vi "InitRegisterLambdaSIM.vi"(8 "error in":errorcluster, 10 "value":T1={"Loop time"={"Period [ms]"=5, "Processor"=-2}, "COM"={"COM IP"="192.168.8.70", "COM port"=30005, "Local port"=5556, "Next_IP 1"=0, "Next_IP 2"=0, "Next_IP 3"=0, "Next_IP 4"=0}, "O2Sensor1"={"Lambda"={"LSU4.2 Lambda"=[], "LSU4.2 Ip"=[], "LSU4.9 Lambda"=[], "LSU4.9 Ip"=[], "LZA03 Lambda"=[], "LZA03 Ip"=[], "LZA08 Lambda"=[], "LZA08 Ip"=[], "Custom Lambda"=[], "Custom Ip"=[]}, "Temp"={"LSU4.2 Temp"=[], "LSU4.2 Ohm"=[], "LSU4.9 Temp"=[], "LSU4.9 Ohm"=[], "LZA03 Temp"=[], "LZA03 Ohm"=[], "LZA08 Temp"=[], "LZA08 Ohm"=[], "Custom Temp"=[], "Custom Ohm"=[]}, "Lambda Type"=0, "PID"={"Ki"=0.0, "Kp"=0.0, "Kd"=0.0, "FeedFW"=0.0}}, "O2Sensor2"={"Lambda"={"LSU4.2 Lambda"=[], "LSU4.2 Ip"=[], "LSU4.9 Lambda"=[], "LSU4.9 Ip"=[], "LZA03 Lambda"=[], "LZA03 Ip"=[], "LZA08 Lambda"=[], "LZA08 Ip"=[], "Custom Lambda"=[], "Custom Ip"=[]}, "Temp"={"LSU4.2 Temp"=[], "LSU4.2 Ohm"=[], "LSU4.9 Temp"=[], "LSU4.9 Ohm"=[], "LZA03 Temp"=[], "LZA03 Ohm"=[], "LZA08 Temp"=[], "LZA08 Ohm"=[], "Custom Temp"=[], "Custom Ohm"=[]}, "Lambda Type"=0, "PID"={"Ki"=0.0, "Kp"=0.0, "Kd"=0.0, "FeedFW"=0.0}}, "O2Sensor3"={"Lambda"={"LSU4.2 Lambda"=[], "LSU4.2 Ip"=[], "LSU4.9 Lambda"=[], "LSU4.9 Ip"=[], "LZA03 Lambda"=[], "LZA03 Ip"=[], "LZA08 Lambda"=[], "LZA08 Ip"=[], "Custom Lambda"=[], "Custom Ip"=[]}, "Temp"={"LSU4.2 Temp"=[], "LSU4.2 Ohm"=[], "LSU4.9 Temp"=[], "LSU4.9 Ohm"=[], "LZA03 Temp"=[], "LZA03 Ohm"=[], "LZA08 Temp"=[], "LZA08 Ohm"=[], "Custom Temp"=[], "Custom Ohm"=[]}, "Lambda Type"=0, "PID"={"Ki"=0.0, "Kp"=0.0, "Kd"=0.0, "FeedFW"=0.0}}, "O2Sensor4"={"Lambda"={"LSU4.2 Lambda"=[], "LSU4.2 Ip"=[], "LSU4.9 Lambda"=[], "LSU4.9 Ip"=[], "LZA03 Lambda"=[], "LZA03 Ip"=[], "LZA08 Lambda"=[], "LZA08 Ip"=[], "Custom Lambda"=[], "Custom Ip"=[]}, "Temp"={"LSU4.2 Temp"=[], "LSU4.2 Ohm"=[], "LSU4.9 Temp"=[], "LSU4.9 Ohm"=[], "LZA03 Temp"=[], "LZA03 Ohm"=[], "LZA08 Temp"=[], "LZA08 Ohm"=[], "Custom Temp"=[], "Custom Ohm"=[]}, "Lambda Type"=0, "PID"={"Ki"=0.0, "Kp"=0.0, "Kd"=0.0, "FeedFW"=0.0}}, "Board"=0, "Mode"=enum."SLSC Mode", "vendor.Num"=4141, "product.Num"=0} {"Board" items=["O2Sim_2ch", "O2Sim_4ch"]; "O2Sensor4"."Lambda Type" items=["LSU4.2", "LSU4.9", "LZA03", "LZA08", "Custom", "[mA]"]; "O2Sensor3"."Lambda Type" items=["LSU4.2", "LSU4.9", "LZA03", "LZA08", "Custom", "[mA]"]; "O2Sensor2"."Lambda Type" items=["LSU4.2", "LSU4.9", "LZA03", "LZA08", "Custom", "[mA]"]; "O2Sensor1"."Lambda Type" items=["LSU4.2", "LSU4.9", "LZA03", "LZA08", "Custom", "[mA]"]}, 11 "session in":refnum<k21>) -> (0 "error out":errorcluster, 2 "COM error":bool, 3 "session out":refnum<k21>)   [LabVIEW 2017, in "ALMA_10201-10401_O2SensorSim Engine.lvlib"]
uses:
  ALMA_10201-10401_O2SensorSim Engine.lvlib
  Par.ctl
  LambdaType.ctl
  <vilib>/SLSC/Write Register (U64).vi
  <vilib>/SLSC/Read Register (U64).vi
  <vilib>/SLSC/SLSC.lvlib
panel:
  out "x = y?":bool
  out "CommandCounter":u8
  out "COM error0":bool
  out "IP Feedback 7":dbl[](array[numeric])
  out "Command Cunter Feedback 7":u8=255
  out "Program Running Cunter 7":u8=96
  in  "CommandData 7":u64 format="%048b"
  out "IP Feedback 4":dbl[](array[numeric])
  out "Command Cunter Feedback 4":u8=255
  out "Program Running Cunter 4":u8=96
  in  "CommandData 5":u64 format="%048b"
  out "IP Feedback 3":dbl[](array[numeric])
  out "Command Cunter Feedback 3":u8=255
  out "Program Running Cunter 3":u8=96
  in  "CommandData 3":u64 format="%048b"
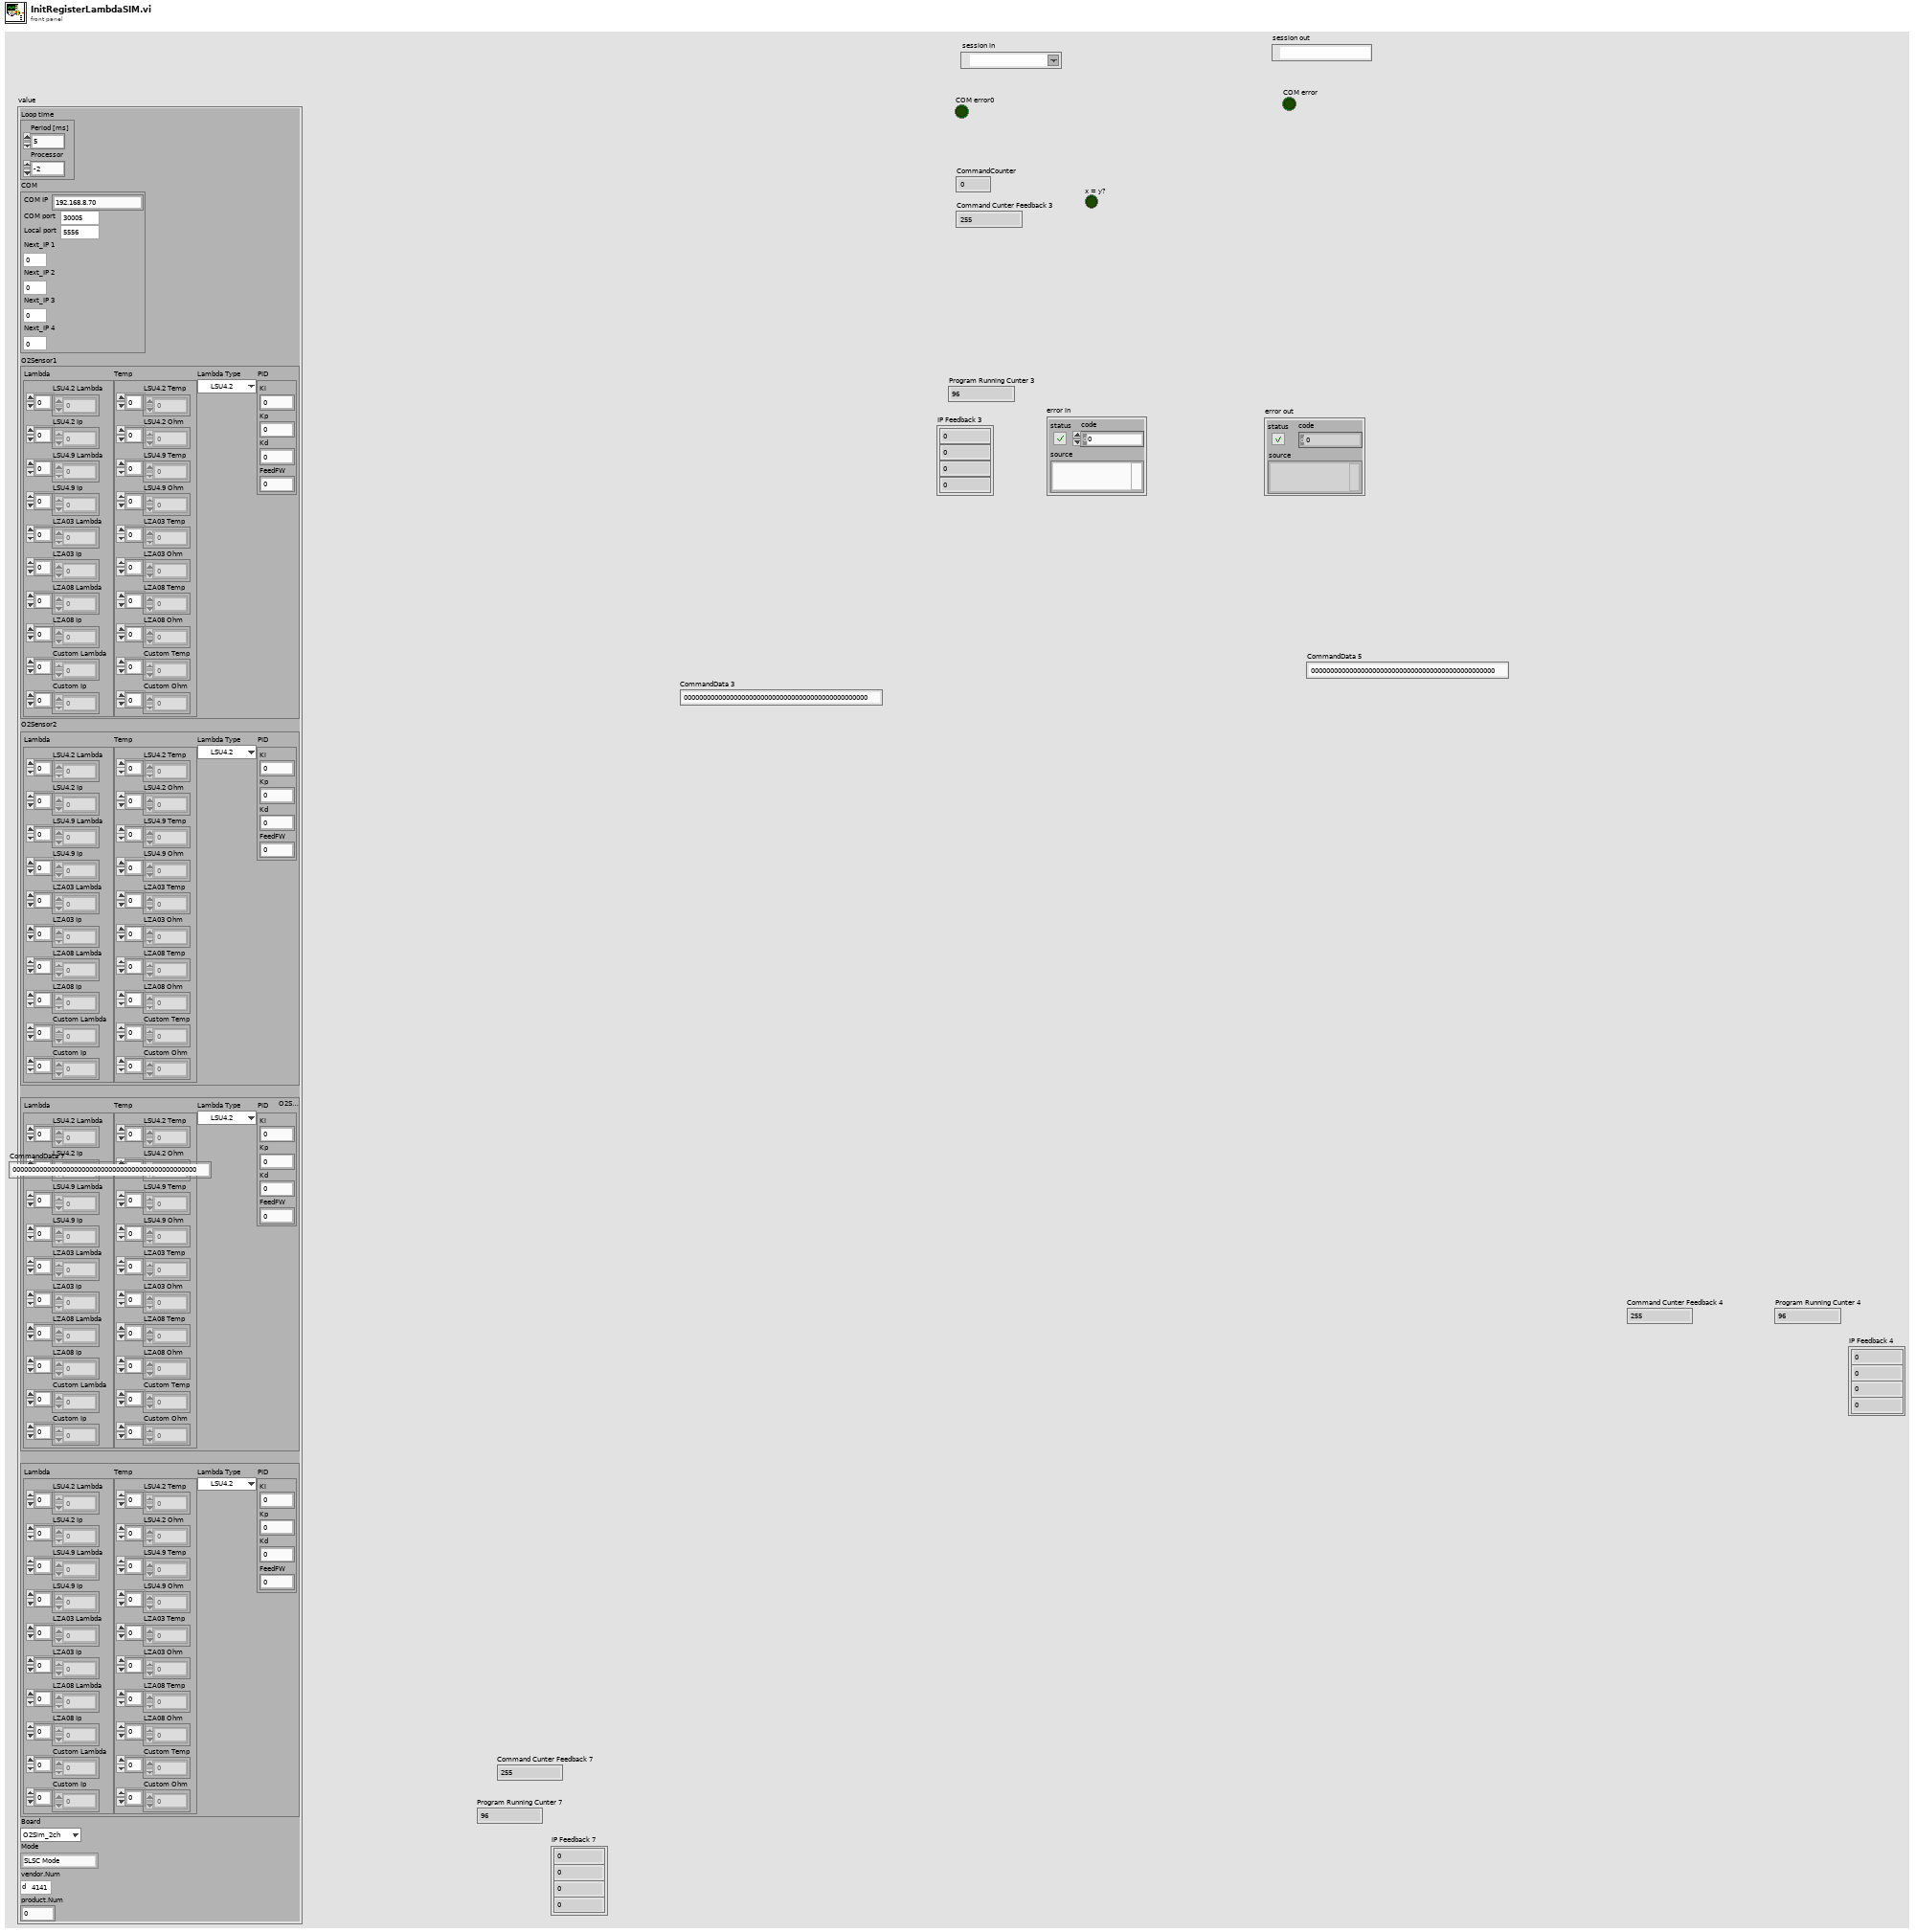
[diagram p1: front panel]
types:
  T1 = typedef "Par.ctl" = cluster{"Loop time":cluster{"Period [ms]":i64, "Processor":i32}, "COM":cluster{"COM IP":string, "COM port":u64, "Local port":u64, "Next_IP 1":u32, "Next_IP 2":u32, "Next_IP 3":u32, "Next_IP 4":u32}, "O2Sensor1":cluster{"Lambda":cluster{"LSU4.2 Lambda":dbl[], "LSU4.2 Ip":dbl[], "LSU4.9 Lambda":dbl[], "LSU4.9 Ip":dbl[], "LZA03 Lambda":dbl[], "LZA03 Ip":dbl[], "LZA08 Lambda":dbl[], "LZA08 Ip":dbl[], "Custom Lambda":dbl[], "Custom Ip":dbl[]}, "Temp":cluster{"LSU4.2 Temp":dbl[], "LSU4.2 Ohm":dbl[], "LSU4.9 Temp":dbl[], "LSU4.9 Ohm":dbl[], "LZA03 Temp":dbl[], "LZA03 Ohm":dbl[], "LZA08 Temp":dbl[], "LZA08 Ohm":dbl[], "Custom Temp":dbl[], "Custom Ohm":dbl[]}, "Lambda Type":T2, "PID":cluster{"Ki":dbl, "Kp":dbl, "Kd":dbl, "FeedFW":dbl}}, "O2Sensor2":cluster{"Lambda":cluster{"LSU4.2 Lambda":dbl[], "LSU4.2 Ip":dbl[], "LSU4.9 Lambda":dbl[], "LSU4.9 Ip":dbl[], "LZA03 Lambda":dbl[], "LZA03 Ip":dbl[], "LZA08 Lambda":dbl[], "LZA08 Ip":dbl[], "Custom Lambda":dbl[], "Custom Ip":dbl[]}, "Temp":cluster{"LSU4.2 Temp":dbl[], "LSU4.2 Ohm":dbl[], "LSU4.9 Temp":dbl[], "LSU4.9 Ohm":dbl[], "LZA03 Temp":dbl[], "LZA03 Ohm":dbl[], "LZA08 Temp":dbl[], "LZA08 Ohm":dbl[], "Custom Temp":dbl[], "Custom Ohm":dbl[]}, "Lambda Type":T2, "PID":cluster{"Ki":dbl, "Kp":dbl, "Kd":dbl, "FeedFW":dbl}}, "O2Sensor3":cluster{"Lambda":cluster{"LSU4.2 Lambda":dbl[], "LSU4.2 Ip":dbl[], "LSU4.9 Lambda":dbl[], "LSU4.9 Ip":dbl[], "LZA03 Lambda":dbl[], "LZA03 Ip":dbl[], "LZA08 Lambda":dbl[], "LZA08 Ip":dbl[], "Custom Lambda":dbl[], "Custom Ip":dbl[]}, "Temp":cluster{"LSU4.2 Temp":dbl[], "LSU4.2 Ohm":dbl[], "LSU4.9 Temp":dbl[], "LSU4.9 Ohm":dbl[], "LZA03 Temp":dbl[], "LZA03 Ohm":dbl[], "LZA08 Temp":dbl[], "LZA08 Ohm":dbl[], "Custom Temp":dbl[], "Custom Ohm":dbl[]}, "Lambda Type":T2, "PID":cluster{"Ki":dbl, "Kp":dbl, "Kd":dbl, "FeedFW":dbl}}, "O2Sensor4":cluster{"Lambda":cluster{"LSU4.2 Lambda":dbl[], "LSU4.2 Ip":dbl[], "LSU4.9 Lambda":dbl[], "LSU4.9 Ip":dbl[], "LZA03 Lambda":dbl[], "LZA03 Ip":dbl[], "LZA08 Lambda":dbl[], "LZA08 Ip":dbl[], "Custom Lambda":dbl[], "Custom Ip":dbl[]}, "Temp":cluster{"LSU4.2 Temp":dbl[], "LSU4.2 Ohm":dbl[], "LSU4.9 Temp":dbl[], "LSU4.9 Ohm":dbl[], "LZA03 Temp":dbl[], "LZA03 Ohm":dbl[], "LZA08 Temp":dbl[], "LZA08 Ohm":dbl[], "Custom Temp":dbl[], "Custom Ohm":dbl[]}, "Lambda Type":T2, "PID":cluster{"Ki":dbl, "Kp":dbl, "Kd":dbl, "FeedFW":dbl}}, "Board":u16, "Mode":enum16{"SLSC Mode", "ANALOG Mode"}, "vendor.Num":u32, "product.Num":u32}
  T2 = typedef "LambdaType.ctl" = u16
  T3 = cluster{"Lambda":cluster{"LSU4.2 Lambda":dbl[], "LSU4.2 Ip":dbl[], "LSU4.9 Lambda":dbl[], "LSU4.9 Ip":dbl[], "LZA03 Lambda":dbl[], "LZA03 Ip":dbl[], "LZA08 Lambda":dbl[], "LZA08 Ip":dbl[], "Custom Lambda":dbl[], "Custom Ip":dbl[]}, "Temp":cluster{"LSU4.2 Temp":dbl[], "LSU4.2 Ohm":dbl[], "LSU4.9 Temp":dbl[], "LSU4.9 Ohm":dbl[], "LZA03 Temp":dbl[], "LZA03 Ohm":dbl[], "LZA08 Temp":dbl[], "LZA08 Ohm":dbl[], "Custom Temp":dbl[], "Custom Ohm":dbl[]}, "Lambda Type":T2, "PID":cluster{"Ki":dbl, "Kp":dbl, "Kd":dbl, "FeedFW":dbl}}
  T4 = cluster{"Lambda":cluster{"LSU4.2 Lambda":dbl[], "LSU4.2 Ip":dbl[], "LSU4.9 Lambda":dbl[], "LSU4.9 Ip":dbl[], "LZA03 Lambda":dbl[], "LZA03 Ip":dbl[], "LZA08 Lambda":dbl[], "LZA08 Ip":dbl[], "Custom Lambda":dbl[], "Custom Ip":dbl[]}, "Temp":cluster{"LSU4.2 Temp":dbl[], "LSU4.2 Ohm":dbl[], "LSU4.9 Temp":dbl[], "LSU4.9 Ohm":dbl[], "LZA03 Temp":dbl[], "LZA03 Ohm":dbl[], "LZA08 Temp":dbl[], "LZA08 Ohm":dbl[], "Custom Temp":dbl[], "Custom Ohm":dbl[]}, "Lambda Type":T2, "PID":cluster{"Ki":dbl, "Kp":dbl, "Kd":dbl, "FeedFW":dbl}}[]
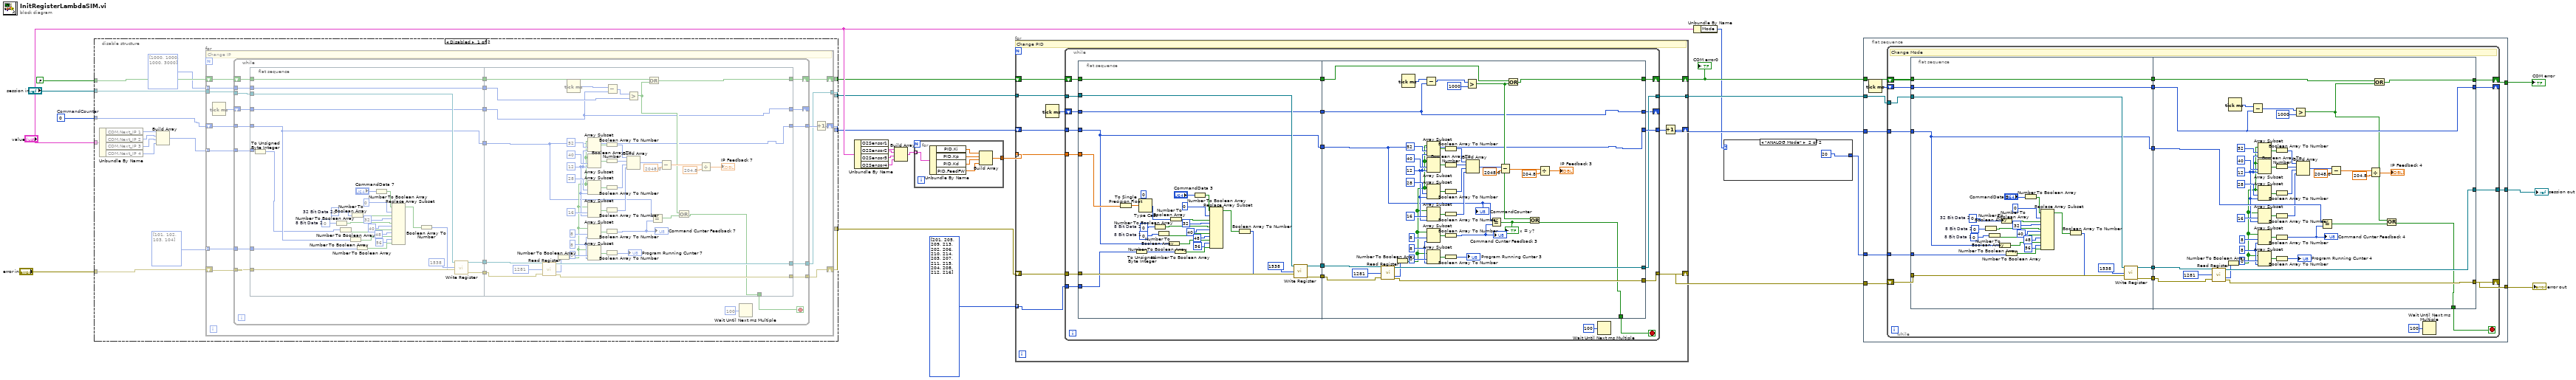
[diagram p0: block diagram]
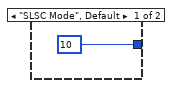
[diagram p3: hidden frame]
diagram:
  w1 = u8 0  # CommandCounter
  n1 = disable-structure shown="Disabled" {
    disable-tunnel: "value" -> [w41 _]
    disable-tunnel: "session in" -> [w40 w148]
    disable-tunnel: "error in" -> [w34 w147]
    disable-tunnel: FALSE -> [w33 w149]
    disable-tunnel: [w30 w148] -> w11
    disable-tunnel: [w29 w149] -> w10
    disable-tunnel: [w28 w146] -> w9
    disable-tunnel: [w27 w147] -> w6
    disable-tunnel: w1 -> [w26 w146]
    frame Disabled {
      n2 = Unbundle By Name(w41) -> ("COM.Next_IP 1"=w39:u32, "COM.Next_IP 2"=w38:u32, "COM.Next_IP 3"=w37:u32, "COM.Next_IP 4"=w32:u32)
      n3 = Build Array(w39, w38, w37, w32) -> (w36:u32[])
      n4 = for {
        tunnel: w40 -> [w54]
        tunnel: w36 -> [w53] mode=indexing
        tunnel: u8[] [101, 102, 103, 104] -> [w52] mode=indexing
        shift-right: [w42] -> w28
        shift-left: w26 -> [w51]
        shift-right: [w49] -> w27
        shift-left: w34 -> [w48]
        tunnel: [w47] -> w30
        shift-right: [w45] -> w29
        shift-left: w33 -> [w44]
        tunnel: u32[] [1000, 1000, 1000, 3000] -> [w43] mode=indexing
        # "Change IP"
        n5 = Tick Count (ms)() -> (millisecond timer value=w46:u32)
        n6 = while {
          tunnel: w54 -> [w72]
          tunnel: w53 -> [w71]
          tunnel: w52 -> [w70]
          tunnel: w51 -> [w69]
          tunnel: [w68] -> w50
          tunnel: [w67] -> w49
          tunnel: w48 -> [w66]
          tunnel: [w65] -> w47
          shift-right: [w62] -> _
          shift-left: w46 -> [w63]
          shift-right: [w60] -> w45
          shift-left: w44 -> [w58]
          tunnel: w43 -> [w57]
          stop <- w61 stop-if-true
          n7 = flat-sequence {
            tunnel: w66 -> [w102]
            tunnel: w72 -> [w101]
            tunnel: [w85] -> w75
            tunnel: [w84] -> w74
            tunnel: [w82] -> w73
            tunnel: w71 -> [w77]
            tunnel: w70 -> [w83]
            tunnel: w69 -> [w82]
            tunnel: [w81] -> w64
            tunnel: w63 -> [w81]
            tunnel: [w80] -> w59
            tunnel: w58 -> [w80]
            tunnel: w57 -> [w79]
            tunnel: [w79] -> w56
            tunnel: w75 -> [w145]
            tunnel: w74 -> [w144]
            tunnel: w73 -> [w105]
            tunnel: [w105] -> w68
            tunnel: [w143] -> w67
            tunnel: [w142] -> w65
            tunnel: w64 -> [w104]
            tunnel: [w104] -> w62
            tunnel: [w107] -> w61
            tunnel: [w110] -> w60
            tunnel: w59 -> [w111]
            tunnel: w56 -> [w109]
            frame #0 {
              w78 = u32 0  # 32 Bit Data 2
              w88 = u8 0  # 8 Bit Data 2
              n8 = To Unsigned Byte Integer(number=w77) -> (unsigned 8bit integer=w76:u8)
              n9 = Number To Boolean Array(number=w88) -> (Boolean array=w86:bool[])
              n10 = Number To Boolean Array(number=w76) -> (Boolean array=w87:bool[])
              n11 = Number To Boolean Array(number=w82) -> (Boolean array=w90:bool[])
              n12 = Number To Boolean Array(number=w78) -> (Boolean array=w89:bool[])
              n13 = Number To Boolean Array(number=w83) -> (Boolean array=w97:bool[])
              n14 = Number To Boolean Array(number="CommandData 7") -> (Boolean array=w99:bool[])
              n15 = Replace Array Subset(array=w99, new element #1=w89, index #1=0 ("index"), new element #2=w86, index #2=32 ("index"), new element #3=w87, index #3=40 ("index"), new element #4=w90, index #4=48 ("index"), new element #5=w97, index #5=56 ("index")) -> (w98:bool[])
              n16 = Boolean Array To Number(Boolean array=w98) -> (number=w94:u64)
              n17 = call-poly <vilib>:"Write Register.vi"("session in"=w101, "register address"=u32 1538, "data"=w94, "error in (no error)"=w102) -> ("session out"=w84:refnum<k21>, "error out"=w85:errorcluster)  [unwired: 8 in, 2 out]
            }
            frame #1 {
              w133 = 8 ("length")
              w134 = 12 ("length")
              n18 = call-poly <vilib>:"Read Register.vi"("session in"=w144, "register address"=u32 1281 ("y"), "error in (no error)"=w145) -> ("session out"=w142:refnum<k21>, "data out"=w115:u64, "error out"=w143:errorcluster)  [unwired: 8 in, 2 out]
              n19 = Number To Boolean Array(number=w115) -> (Boolean array=w128:bool[])
              n20 = Tick Count (ms)() -> (millisecond timer value=w106:u32)
              n21 = Array Subset(array=w128, index=52, length=w134) -> (w129:bool[])
              n22 = Array Subset(array=w128, index=40, length=w134) -> (w127:bool[])
              n23 = Array Subset(array=w128, index=28, length=w134) -> (w126:bool[])
              n24 = Array Subset(array=w128, index=16, length=w134) -> (w125:bool[])
              n25 = Array Subset(array=w128, index=8, length=w133) -> (w124:bool[])
              n26 = Array Subset(array=w128, index=0, length=w133) -> (w123:bool[])
              n27 = Boolean Array To Number(Boolean array=w129) -> (number=w117:u16)
              n28 = Boolean Array To Number(Boolean array=w127) -> (number=w132:u16)
              n29 = Boolean Array To Number(Boolean array=w126) -> (number=w131:u16)
              n30 = Boolean Array To Number(Boolean array=w125) -> (number=w130:u16)
              n31 = Boolean Array To Number(Boolean array=w124) -> (number=w114:u8)
              "Command Cunter Feedback 7" <- w114
              n32 = Boolean Array To Number(Boolean array=w123) -> (number=→"Program Running Cunter 7":u8)
              n33 = Subtract(x=w106, y=w104) -> (x-y=w113:u32)
              n34 = Greater?(x=w113, y=w109) -> (0:w108:bool)
              n35 = Build Array(w117, w132, w131, w130) -> (w118:u16[])
              n36 = Or(x=w111, y=w108) -> (x .or. y?=w110:bool)
              n37 = Equal?(x=w105, y=w114) -> (x = y?=w112:bool)
              n38 = Subtract(x=w118, y=2048.0) -> (x-y=w121:dbl[])
              n39 = Or(x=w108, y=w112) -> (x .or. y?=w107:bool)
              n40 = Divide(x=w121, y=204.8) -> (x/y=→"IP Feedback 7":dbl[])
            }
          }
          n41 = Wait Until Next ms Multiple(millisecond multiple=u32 100) -> ()  [unwired: 1 out]
        }
        n42 = Increment(x=w50) -> (x+1=w42:u8)
      }
    }
    frame Enabled {
    }
  }
  n43 = Unbundle By Name("value") -> ("O2Sensor1"=w25:T3, "O2Sensor2"=w24:T3, "O2Sensor3"=w23:T3, "O2Sensor4"=w22:T3)
  n44 = Build Array(w25, w24, w23, w22) -> (w8:T4)
  n45 = for {
    tunnel: w8 -> [w155] mode=indexing
    tunnel: [w150] -> w7 mode=concatenating
    n46 = Unbundle By Name(w155) -> ("PID.Ki"=w154:dbl, "PID.Kp"=w153:dbl, "PID.Kd"=w152:dbl, "PID.FeedFW"=w151:dbl)
    n47 = Build Array(w154, w153, w152, w151) -> (w150:dbl[])
  }
  n48 = for {
    tunnel: w11 -> [w167]
    tunnel: w7 -> [w166] mode=indexing
    shift-right: [w157] -> w20
    shift-left: w9 -> [w165]
    shift-right: [w163] -> w19
    shift-left: w6 -> [w162]
    tunnel: [w161] -> w21
    shift-right: [w158] -> w5
    shift-left: w10 -> [w160]
    tunnel: u8[] [201, 205, 209, 213, 202, 206, 210, 214, 203, 207, 211, 215, 204, 208, 212, 216] -> [w156] mode=indexing
    # "Change PID"
    n49 = Tick Count (ms)() -> (millisecond timer value=w159:u32)
    n50 = while {
      tunnel: w166 -> [w182]
      tunnel: w165 -> [w181]
      tunnel: [w180] -> w164
      tunnel: [w179] -> w163
      tunnel: w162 -> [w178]
      shift-right: [w172] -> _
      shift-left: w159 -> [w175]
      shift-right: [w170] -> w158
      shift-left: w160 -> [w176]
      tunnel: w156 -> [w169]
      tunnel: w167 -> [w183]
      tunnel: [w177] -> w161
      stop <- w173 stop-if-true
      n51 = flat-sequence {
        tunnel: w178 -> [w215]
        tunnel: w183 -> [w214]
        tunnel: [w194] -> w186
        tunnel: [w193] -> w185
        tunnel: [w191] -> w184
        tunnel: w182 -> [w192]
        tunnel: w181 -> [w191]
        tunnel: w176 -> [w189]
        tunnel: w175 -> [w190]
        tunnel: [w190] -> w174
        tunnel: [w189] -> w171
        tunnel: w169 -> [w188]
        tunnel: w186 -> [w258]
        tunnel: w185 -> [w257]
        tunnel: w184 -> [w218]
        tunnel: [w218] -> w180
        tunnel: [w256] -> w179
        tunnel: [w255] -> w177
        tunnel: w174 -> [w217]
        tunnel: [w223] -> w173
        tunnel: [w217] -> w172
        tunnel: w171 -> [w221]
        tunnel: [w219] -> w170
        frame #0 {
          w197 = u8 0  # 8 Bit Data 2
          w198 = u8 0  # 8 Bit Data 1
          n52 = To Single Precision Float(number=w192) -> (single precision float=w206:sgl)
          n53 = To Unsigned Byte Integer(number=w188) -> (unsigned 8bit integer=w187:u8)
          n54 = Type Cast(type=u32 0 ("index"), x=w206) -> (*(type *) &x=w199:u32)
          n55 = Number To Boolean Array(number=w197) -> (Boolean array=w195:bool[])
          n56 = Number To Boolean Array(number=w198) -> (Boolean array=w196:bool[])
          n57 = Number To Boolean Array(number=w191) -> (Boolean array=w201:bool[])
          n58 = Number To Boolean Array(number=w199) -> (Boolean array=w200:bool[])
          n59 = Number To Boolean Array(number=w187) -> (Boolean array=w210:bool[])
          n60 = Number To Boolean Array(number="CommandData 3") -> (Boolean array=w212:bool[])
          n61 = Replace Array Subset(array=w212, new element #1=w200, index #1=0 ("index"), new element #2=w195, index #2=32 ("index"), new element #3=w196, index #3=40 ("index"), new element #4=w201, index #4=48 ("index"), new element #5=w210, index #5=56 ("index")) -> (w211:bool[])
          n62 = Boolean Array To Number(Boolean array=w211) -> (number=w207:u64)
          n63 = call-poly <vilib>:"Write Register.vi"("session in"=w214, "register address"=u32 1538, "data"=w207, "error in (no error)"=w215) -> ("session out"=w193:refnum<k21>, "error out"=w194:errorcluster)  [unwired: 8 in, 2 out]
        }
        frame #1 {
          w246 = 8 ("length")
          w247 = 12 ("length")
          n64 = call-poly <vilib>:"Read Register.vi"("session in"=w257, "register address"=u32 1281 ("y"), "error in (no error)"=w258) -> ("session out"=w255:refnum<k21>, "data out"=w228:u64, "error out"=w256:errorcluster)  [unwired: 8 in, 2 out]
          n65 = Number To Boolean Array(number=w228) -> (Boolean array=w241:bool[])
          n66 = Tick Count (ms)() -> (millisecond timer value=w222:u32)
          n67 = Subtract(x=w222, y=w217) -> (x-y=w225:u32)
          n68 = Array Subset(array=w241, index=52, length=w247) -> (w242:bool[])
          n69 = Array Subset(array=w241, index=40, length=w247) -> (w240:bool[])
          n70 = Array Subset(array=w241, index=28, length=w247) -> (w239:bool[])
          n71 = Array Subset(array=w241, index=16, length=w247) -> (w238:bool[])
          n72 = Array Subset(array=w241, index=8, length=w246) -> (w237:bool[])
          n73 = Array Subset(array=w241, index=0, length=w246) -> (w236:bool[])
          n74 = Boolean Array To Number(Boolean array=w242) -> (number=w230:u16)
          n75 = Boolean Array To Number(Boolean array=w240) -> (number=w245:u16)
          n76 = Boolean Array To Number(Boolean array=w239) -> (number=w244:u16)
          n77 = Boolean Array To Number(Boolean array=w238) -> (number=w243:u16)
          n78 = Boolean Array To Number(Boolean array=w237) -> (number=w227:u8)
          "Command Cunter Feedback 3" <- w227
          n79 = Boolean Array To Number(Boolean array=w236) -> (number=→"Program Running Cunter 3":u8)
          n80 = Greater?(x=w225, y=u32 1000) -> (0:w220:bool)
          n81 = Build Array(w230, w245, w244, w243) -> (w231:u16[])
          n82 = Equal?(x=w218, y=w227) -> (x = y?=w226:bool)
          "x = y?" <- w226
          n83 = Subtract(x=w231, y=2048.0) -> (x-y=w234:dbl[])
          n84 = Or(x=w221, y=w220) -> (x .or. y?=w219:bool)
          n85 = Or(x=w220, y=w226) -> (x .or. y?=w223:bool)
          n86 = Divide(x=w234, y=204.8) -> (x/y=→"IP Feedback 3":dbl[])
          "CommandCounter" <- w218
        }
      }
      n87 = Wait Until Next ms Multiple(millisecond multiple=u32 100) -> ()  [unwired: 1 out]
    }
    n88 = Increment(x=w164) -> (x+1=w157:u8)
  }
  "COM error0" <- w5
  n89 = Unbundle By Name("value") -> ("Mode"=w2:enum16{"SLSC Mode", "ANALOG Mode"})
  n90 = case shown="\"ANALOG Mode\"" w2 {
    tunnel: [u8 10 ("CommandWord") u8 20 ("CommandWord")] -> w16
    frame "SLSC Mode", Default {
    }
    frame "ANALOG Mode" {
    }
  }
  n91 = flat-sequence {
    tunnel: w21 -> [w269]
    tunnel: w20 -> [w268]
    tunnel: w19 -> [w267]
    tunnel: [w266] -> w18
    tunnel: [w265] -> w17
    tunnel: w16 -> [w264]
    tunnel: w5 -> [w263]
    tunnel: [w261] -> w4
    frame #0 {
      n92 = Tick Count (ms)() -> (millisecond timer value=w262:u32)
      n93 = while {
        tunnel: w268 -> [w282]
        tunnel: w264 -> [w278]
        shift-right: [w279] -> w265
        shift-left: w267 -> [w281]
        tunnel: w269 -> [w283]
        tunnel: [w280] -> w266
        shift-right: [w271] -> w261
        shift-left: w263 -> [w277]
        shift-right: [w273] -> _
        shift-left: w262 -> [w275]
        stop <- w276 stop-if-true
        # "Change Mode"
        n94 = flat-sequence {
          tunnel: w281 -> [w311]
          tunnel: w283 -> [w310]
          tunnel: [w293] -> w286
          tunnel: [w292] -> w285
          tunnel: [w290] -> w284
          tunnel: w278 -> [w291]
          tunnel: w282 -> [w290]
          tunnel: w277 -> [w287]
          tunnel: w275 -> [w288]
          tunnel: [w288] -> w274
          tunnel: [w287] -> w272
          tunnel: w286 -> [w354]
          tunnel: w285 -> [w353]
          tunnel: w284 -> [w352]
          tunnel: [w351] -> w279
          tunnel: [w350] -> w280
          tunnel: [w317] -> w276
          tunnel: w274 -> [w316]
          tunnel: [w316] -> w273
          tunnel: w272 -> [w315]
          tunnel: [w314] -> w271
          frame #0 {
            w289 = u32 0  # 32 Bit Data 2
            w296 = u8 0  # 8 Bit Data 2
            w297 = u8 0  # 8 Bit Data 1
            n95 = Number To Boolean Array(number=w296) -> (Boolean array=w294:bool[])
            n96 = Number To Boolean Array(number=w297) -> (Boolean array=w295:bool[])
            n97 = Number To Boolean Array(number=w290) -> (Boolean array=w299:bool[])
            n98 = Number To Boolean Array(number=w289) -> (Boolean array=w298:bool[])
            n99 = Number To Boolean Array(number=w291) -> (Boolean array=w306:bool[])
            n100 = Number To Boolean Array(number="CommandData 5") -> (Boolean array=w308:bool[])
            n101 = Replace Array Subset(array=w308, new element #1=w298, index #1=0 ("index"), new element #2=w294, index #2=32 ("index"), new element #3=w295, index #3=40 ("index"), new element #4=w299, index #4=48 ("index"), new element #5=w306, index #5=56 ("index")) -> (w307:bool[])
            n102 = Boolean Array To Number(Boolean array=w307) -> (number=w303:u64)
            n103 = call-poly <vilib>:"Write Register.vi"("session in"=w310, "register address"=u32 1538, "data"=w303, "error in (no error)"=w311) -> ("session out"=w292:refnum<k21>, "error out"=w293:errorcluster)  [unwired: 8 in, 2 out]
          }
          frame #1 {
            w341 = 8 ("length")
            w342 = 12 ("length")
            n104 = call-poly <vilib>:"Read Register.vi"("session in"=w353, "register address"=u32 1281 ("y"), "error in (no error)"=w354) -> ("session out"=w350:refnum<k21>, "data out"=w323:u64, "error out"=w351:errorcluster)  [unwired: 8 in, 2 out]
            n105 = Number To Boolean Array(number=w323) -> (Boolean array=w336:bool[])
            n106 = Tick Count (ms)() -> (millisecond timer value=w320:u32)
            n107 = Subtract(x=w320, y=w316) -> (x-y=w319:u32)
            n108 = Array Subset(array=w336, index=52, length=w342) -> (w337:bool[])
            n109 = Array Subset(array=w336, index=40, length=w342) -> (w335:bool[])
            n110 = Array Subset(array=w336, index=28, length=w342) -> (w334:bool[])
            n111 = Array Subset(array=w336, index=16, length=w342) -> (w333:bool[])
            n112 = Array Subset(array=w336, index=8, length=w341) -> (w332:bool[])
            n113 = Array Subset(array=w336, index=0, length=w341) -> (w331:bool[])
            n114 = Boolean Array To Number(Boolean array=w337) -> (number=w325:u16)
            n115 = Boolean Array To Number(Boolean array=w335) -> (number=w340:u16)
            n116 = Boolean Array To Number(Boolean array=w334) -> (number=w339:u16)
            n117 = Boolean Array To Number(Boolean array=w333) -> (number=w338:u16)
            n118 = Boolean Array To Number(Boolean array=w332) -> (number=w322:u8)
            "Command Cunter Feedback 4" <- w322
            n119 = Boolean Array To Number(Boolean array=w331) -> (number=→"Program Running Cunter 4":u8)
            n120 = Greater?(x=w319, y=u32 1000) -> (0:w313:bool)
            n121 = Build Array(w325, w340, w339, w338) -> (w326:u16[])
            n122 = Equal?(x=w352, y=w322) -> (x = y?=w321:bool)
            n123 = Subtract(x=w326, y=2048.0) -> (x-y=w329:dbl[])
            n124 = Divide(x=w329, y=204.8) -> (x/y=→"IP Feedback 4":dbl[])
            n125 = Or(x=w315, y=w313) -> (x .or. y?=w314:bool)
            n126 = Or(x=w313, y=w321) -> (x .or. y?=w317:bool)
          }
        }
        n127 = Wait Until Next ms Multiple(millisecond multiple=u32 100) -> ()  [unwired: 1 out]
      }
    }
  }
  "error out" <- w17
  "session out" <- w18
  "COM error" <- w4
